vi "RT Execution State.vi"(0 "Module ID In":i32, 7 "Exec State?":bool, 11 "error in":errorcluster, 13 "Action":T1) -> (4 "Exec State? Out":bool, 8 "Module ID's":i32[](array[numeric]), 10 "Exec State's?":bool[](array[boolean]), 15 "error out":errorcluster)   [LabVIEW 2019]
uses:
  Host-Control's/RT Exec FGV Action.ctl
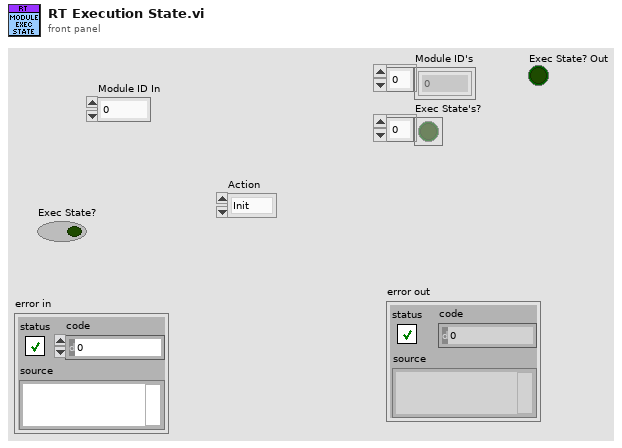
[diagram p1: front panel]
types:
  T1 = typedef "RT Exec FGV Action.ctl" = enum16{"Init", "Insert", "Get a Exec?", "Get All Exec?"}
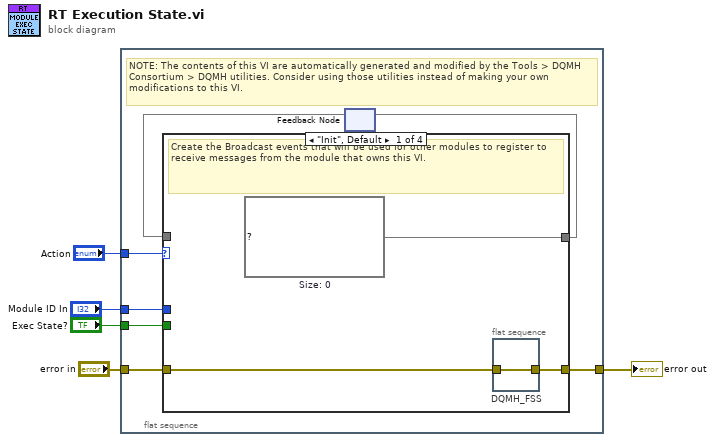
[diagram p0: block diagram]
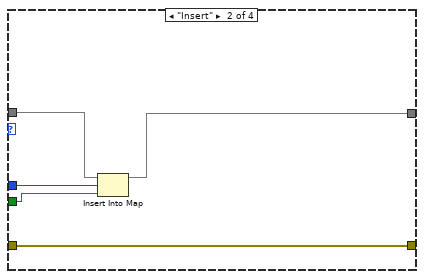
[diagram p2: hidden frame]
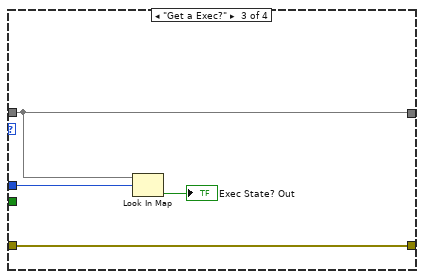
[diagram p3: hidden frame]
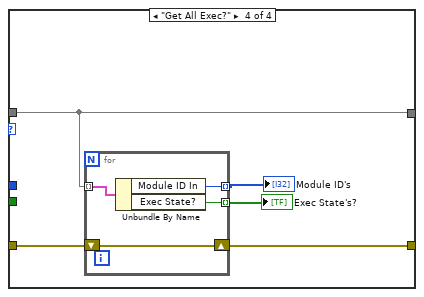
[diagram p4: hidden frame]
diagram:
  n1 = flat-sequence {
    tunnel: [w12] -> w5
    tunnel: "error in" -> [w11]
    tunnel: "Action" -> [w8]
    tunnel: "Module ID In" -> [w7]
    tunnel: "Exec State?" -> [w6]
    frame #0 {
      # "NOTE: The contents of this VI are automatically generated and modified by the Tools > DQMH Consortium > DQMH utilities. Consider using those utilities instead of making your own modifications to this VI."
      n2 = feedback #1() -> (w10:map{i32, bool})  [unwired: 1 in]
      n3 = case shown="\"Init\", Default" w8 {
        tunnel: [w15 w19 w22 w29] -> w12
        tunnel: w11 -> [w14 w19 w22 w28]
        tunnel: [w13 w20 w25 w30] -> w9
        tunnel: w10 -> [_ w21 w25 w30]
        tunnel: w7 -> [_ w18 w24 _]
        tunnel: w6 -> [_ w17 _ _]
        frame "Init", Default {
          w13 = map{i32, bool} {}  # Size: 0
          # "Create the Broadcast events that will be used for other modules to register to receive messages from the module that owns this VI."
          n4 = flat-sequence "DQMH_FSS" {
            tunnel: [w16] -> w15
            tunnel: w14 -> [w16]
            frame #0 {
            }
          }
        }
        frame "Insert" {
          n5 = Insert Into Map(map in=w21, key=w18, value=w17) -> (map out=w20:map{i32, bool})  [unwired: 2 out]
        }
        frame "Get a Exec?" {
          n6 = Look In Map(map=w25, key=w24) -> (value=→"Exec State? Out":bool)  [unwired: 1 in, 1 out]
        }
        frame "Get All Exec?" {
          n7 = for {
            tunnel: w30 -> [w34] mode=indexing
            tunnel: [w33] -> w27 mode=indexing
            tunnel: [w32] -> w26 mode=indexing
            shift-right: [w31] -> w29
            shift-left: w28 -> [w31]
            n8 = Unbundle By Name(w34) -> ("Module ID In"=w33:i32, "Exec State?"=w32:bool)
          }
          "Module ID's" <- w27
          "Exec State's?" <- w26
        }
      }
      n9 = feedback-in #1(w9) -> ()
    }
  }
  "error out" <- w5
